vi "CRYUnflatten Start.vi"(11 "Unflatten Sequence":string) -> (0 "Error?":bool, 2 "Sequence Configure":T1, 3 "Header info":T2={"Data type"="Data            ", "Version"=1, "Dimensions"=0})   [LabVIEW 2013]
uses:
  Typedef Control/CRYStart Cluster.ctl
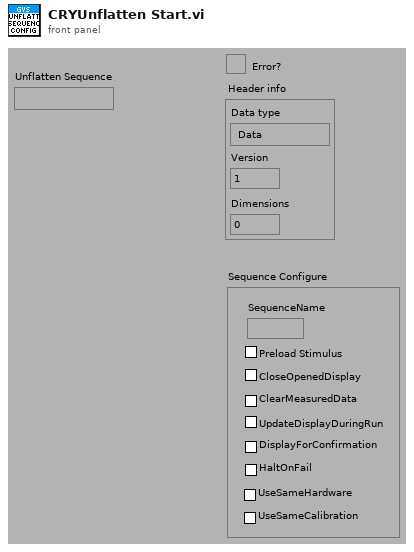
[diagram p1: front panel]
types:
  T1 = typedef "CRYStart Cluster.ctl" = cluster{"SequenceName":string, "Preload Stimulus":bool, "CloseOpenedDisplay":bool, "ClearMeasuredData":bool, "UpdateDisplayDuringRun":bool, "DisplayForConfirmation":bool, "HaltOnFail":bool, "UseSameHardware":bool, "UseSameCalibration":bool}
  T2 = cluster{"Data type":string, "Version":u16, "Dimensions":u8}
  T3 = cluster{"unsigned byte array[0]":u8, "unsigned byte array[1]":u8, "unsigned byte array[2]":u8}
  T4 = cluster{"substring":string, u16, "unsigned byte array[2]":u8}
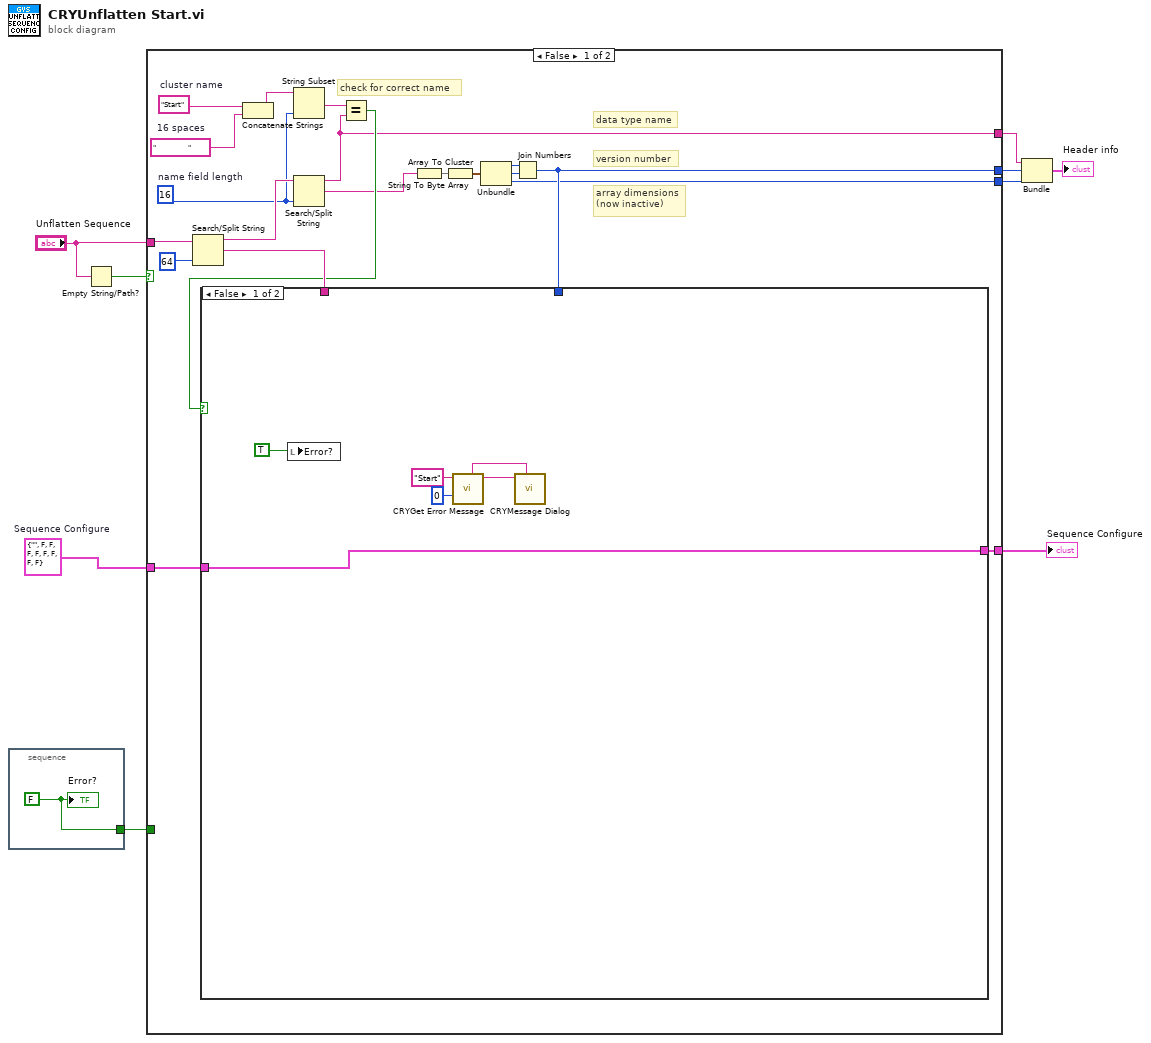
[diagram p0: block diagram]
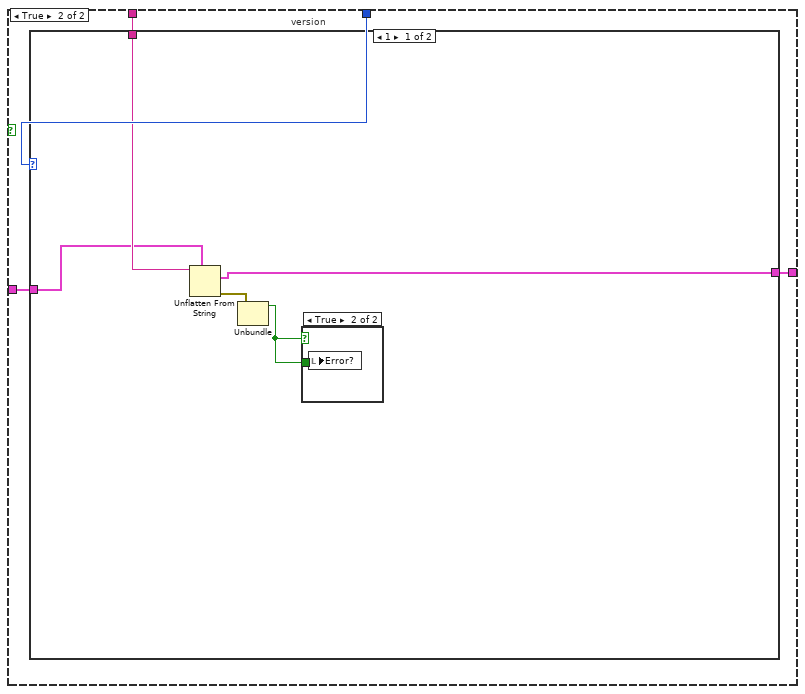
[diagram p2: hidden frame]
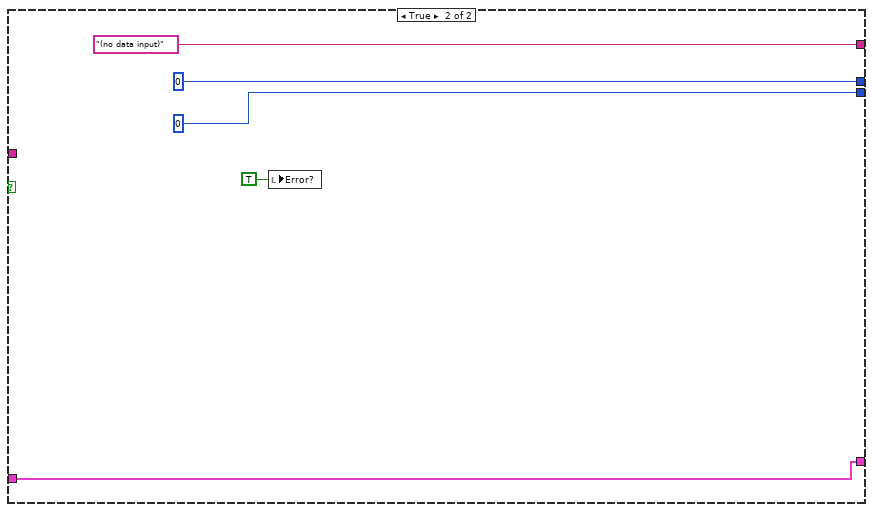
[diagram p5: hidden frame]
diagram:
  w1 = T1 {"SequenceName"="", "Preload Stimulus"=FALSE, "CloseOpenedDisplay"=FALSE, "ClearMeasuredData"=FALSE, "UpdateDisplayDuringRun"=FALSE, "DisplayForConfirmation"=FALSE, "HaltOnFail"=FALSE, "UseSameHardware"=FALSE, "UseSameCalibration"=FALSE}  # Sequence Configure
  n1 = stacked-sequence {
    tunnel: [w10] -> w3
    frame #0 {
      w10 = FALSE
      "Error?" <- w10
    }
  }
  n2 = Empty String/Path?(string/path="Unflatten Sequence") -> (empty?=w8:bool)
  n3 = case shown="False" w8 {
    tunnel: "Unflatten Sequence" -> [w30 _]
    tunnel: [w22 u16 0] -> w6
    tunnel: [w14 u8 0] -> w7
    tunnel: [w15 "(no data input)" ("substring")] -> w5
    tunnel: w3 -> [_ _]
    tunnel: [w13 w48] -> w2
    tunnel: w1 -> [w12 w48]
    frame False {
      w19 = "                "  # 16 spaces
      w20 = "Start"  # cluster name
      w17 = 16  # name field length
      # "check for correct name"
      # "array dimensions\n(now inactive)"
      # "version number"
      # "data type name"
      n4 = Search/Split String(string=w30, offset (0)=64 ("header length")) -> (substring before match=w24:string, match + rest of string=w25:string)  [unwired: 2 out]
      n5 = Concatenate Strings(w20, w19) -> (w18:string)
      n6 = String Subset(string=w18, length (rest)=w17) -> (substring=w16:string)  [unwired: 1 out]
      n7 = Search/Split String(string=w24, offset (0)=w17) -> (substring before match=w15:string, match + rest of string=w21:string)  [unwired: 2 out]
      n8 = Equal?(x=w16, y=w15) -> (x = y?=w23:bool)
      n9 = String To Byte Array(string=w21) -> (unsigned byte array=w29:u8[])
      n10 = Array To Cluster(array=w29) -> (cluster=w28:T3)
      n11 = Unbundle(w28) -> ("unsigned byte array[0]"=w27:u8, "unsigned byte array[1]"=w26:u8, "unsigned byte array[2]"=w14:u8)
      n12 = Join Numbers(hi=w27, lo=w26) -> ((hi.lo)=w22:u16)
      n13 = case shown="False" w23 {
        tunnel: w25 -> [_ w40]
        tunnel: w22 -> [_ w39]
        tunnel: [w35 w38] -> w13
        tunnel: w12 -> [w35 w37]
        frame False {
          n14 = local write "Error?"(TRUE) -> ()
          n15 = call "CRYGet Error Message.vi"("Error No"=0, "Kind"="Start") -> ("Message"=w32:string, "Window Title"=w31:string)  [unwired: 4 in, 4 out]
          n16 = call "CRYMessage Dialog.vi"("Window Title"=w31, "Message Content"=w32) -> ()  [unwired: 8 in, 2 out]
        }
        frame True {
          n17 = case "version" shown="1" w39 {
            tunnel: w40 -> [w45 _]
            tunnel: [w41 w47] -> w38
            tunnel: w37 -> [w42 w47]
            frame 1 {
              n18 = Unflatten From String(type=w42, binary string=w45) -> (value=w41:T1, error out=w43:errorcluster)  [unwired: 1 in, 3 out]
              n19 = Unbundle(w43) -> ("status"=w44:bool)  [unwired: 2 out]
              n20 = case shown="True" w44 {
                tunnel: w44 -> [_ w46]
                frame False {
                }
                frame True {
                  n21 = local write "Error?"(w46) -> ()
                }
              }
            }
            frame Default {
            }
          }
        }
      }
    }
    frame True {
      n22 = local write "Error?"(TRUE ("Error?")) -> ()
    }
  }
  "Sequence Configure" <- w2
  n23 = Bundle("substring"=w5, w6, "unsigned byte array[2]"=w7) -> (→"Header info":T4)  [unwired: 1 out]
